vi "CalcPfundo.vi"(1 "MIN":i32, 2 "MAX":i32=600, 3 "Pbar":dbl, 4 "input":dbl[](array[numeric])) -> (0 "output":dbl[](array[numeric]))   [LabVIEW 2019]
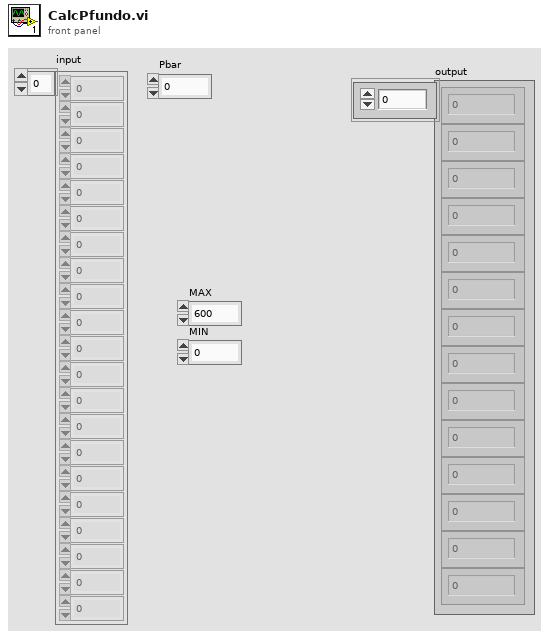
[diagram p1: front panel]
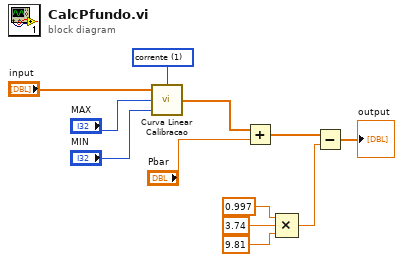
[diagram p0: block diagram]
diagram:
  w11 = u16 1 items=["tensao", "corrente"] ("input type")
  n1 = call "Curva Linear Calibracao.vi"("input type"=w11, "MIN"="MIN", "MAX"="MAX", "input"="input") -> ("output"=w10:dbl[])
  n2 = Add(x=w10, y="Pbar") -> (x+y=w8:dbl[])
  n3 = Compound Arithmetic op=MULTIPLY(0.997, 3.74, 9.81) -> (w4:dbl)
  n4 = Subtract(x=w8, y=w4) -> (x-y=→"output":dbl[])
